vi "computeTurnTarget.vi"(11 "Cluster in":T1) -> (3 "Targpos":sgl[](array[numeric]))   [LabVIEW 2018]
uses:
  TrialListElements.ctl
  trial type.ctl
  rewtype.ctl
  <vilib>/imath/engines/lvmath2/RunTimeEngine/RunTimeType/NIMS_RunTimeType_From StrictType (excl LVString).vi
  <instcachedir>/0/NIMS_RunTimeType_From StrictType (excl LVString)_E7E34A65C99947108168652BAD14964D.lvgen/NIMS_RunTimeType_From StrictType (excl LVString)_E7E34A65C99947108168652BAD14964D_050.vi
  <instcachedir>/0/NIMS_RunTimeType_From StrictType (excl LVString)_E7E34A65C99947108168652BAD14964D.lvgen/NIMS_RunTimeType_From StrictType (excl LVString)_E7E34A65C99947108168652BAD14964D_032.vi
  <instcachedir>/0/NIMS_RunTimeType_From StrictType (excl LVString)_E7E34A65C99947108168652BAD14964D.lvgen/NIMS_RunTimeType_From StrictType (excl LVString)_E7E34A65C99947108168652BAD14964D_031.vi
  <instcachedir>/0/NIMS_RunTimeType_From StrictType (excl LVString)_E7E34A65C99947108168652BAD14964D.lvgen/NIMS_RunTimeType_From StrictType (excl LVString)_E7E34A65C99947108168652BAD14964D_049.vi
  <vilib>/imath/engines/lvmath2/RunTimeEngine/Struct/NIMS_StructSetField.vi
  <vilib>/imath/engines/lvmath2/RunTimeEngine/Struct/NIMS_StructGetField.vi
  <vilib>/imath/engines/lvmath2/RunTimeEngine/RunTimeType/NIMS_RunTimeType_To Numeric.vi
  <instcachedir>/0/NIMS_RunTimeType_To Numeric_56D9B3D2177F45D4A08165E143DC65A4.lvgen/NIMS_RunTimeType_To Numeric_56D9B3D2177F45D4A08165E143DC65A4_008.vi
  <vilib>/imath/engines/lvmath2/RunTimeEngine/IndexReplace/NIMS V(S)=S.vi
  <instcachedir>/0/NIMS V(S)=S_420DA4522869420292A92FA3CC108C4E.lvgen/NIMS V(S)=S_420DA4522869420292A92FA3CC108C4E_000.vi
  <vilib>/imathl/engines/lvmath/Functions/Error Handling/Create Error.vi
  <vilib>/imath/engines/lvmath2/RunTimeEngine/NodeEndStatement/NIMS_NodeEndStatement_Output.vi
  <instcachedir>/0/NIMS_NodeEndStatement_Output_53EC0D466D134D7ABD903AC30B43404B.lvgen/NIMS_NodeEndStatement_Output_53EC0D466D134D7ABD903AC30B43404B_005.vi
  <vilib>/imath/engines/lvmath2/RunTimeEngine/ErrorHandling/NIMS_Finalize Error.vi
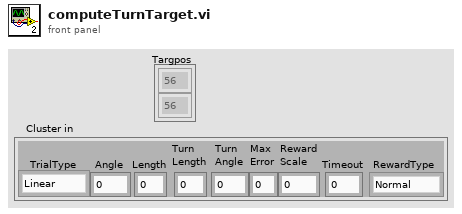
[diagram p1: front panel]
types:
  T1 = typedef "TrialListElements.ctl" = cluster{"TrialType":T2, "Angle":dbl, "Length":dbl, "TurnLength":dbl, "TurnAngle":dbl, "MaxError":dbl, "RewardScale":dbl, "Timeout":i32, "RewardType":T3}
  T2 = typedef "trial type.ctl" = enum8{"Linear", "2D aiming", "Two-part"}
  T3 = typedef "rewtype.ctl" = enum16{"Normal", "No reward"}
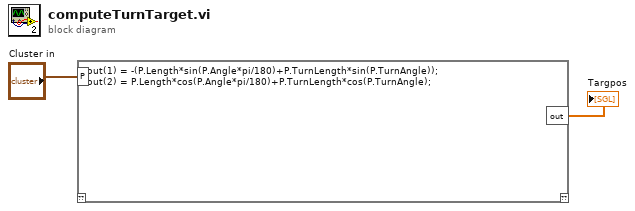
[diagram p0: block diagram]
diagram:
  n1 = mathscript code="out(1) = -(P.Length*sin(P.Angle*pi/180)+P.TurnLength*sin(P.TurnAngle));\nout(2) = P.Length*cos(P.Angle*pi/180)+P.TurnLength*cos(P.TurnAngle);"("P"="Cluster in") -> ("out"=→"Targpos":dbl[])  [unwired: 1 in, 1 out]
